vi "circle center from three points.vi"(9 "z plus":cdb, 10 "z zero":cdb, 11 "z minus":cdb) -> (1 "radius":dbl, 2 "z inf":cdb, 3 "z center":cdb)   [LabVIEW 2015]
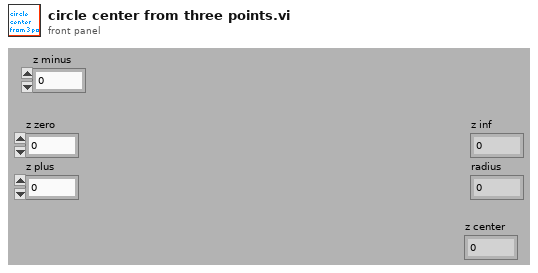
[diagram p1: front panel]
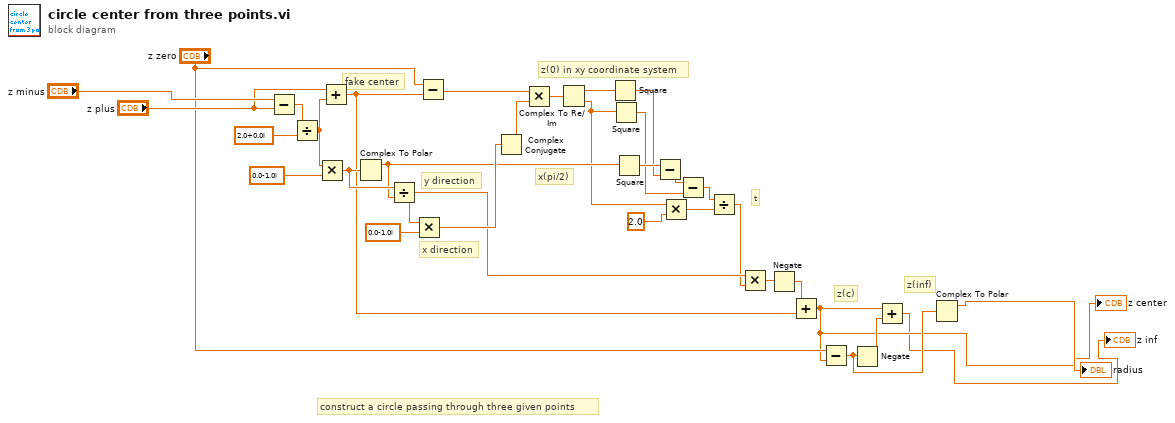
[diagram p0: block diagram]
diagram:
  # "z(inf)"
  # "z(c)"
  # "t"
  # "x(pi/2)"
  # "z(0) in xy coordinate system"
  # "x direction"
  # "y direction"
  # "fake center"
  # "construct a circle passing through three given points"
  n1 = Subtract(x="z minus", y="z plus") -> (x-y=w33:cdb)
  n2 = Divide(x=w33, y=cdb 2.0+0.0i) -> (x/y=w31:cdb)
  n3 = Multiply(x=w31, y=cdb 0.0-1.0i) -> (x*y=w28:cdb)
  n4 = Add(x="z plus", y=w31) -> (x+y=w9:cdb)
  n5 = Complex To Polar(r * e^(i*theta)=w28) -> (r=w23:dbl)  [unwired: 1 out]
  n6 = Divide(x=w28, y=w23) -> (x/y=w13:cdb)
  n7 = Multiply(x=w13, y=cdb 0.0-1.0i) -> (x*y=w27:cdb)
  n8 = Subtract(x="z zero", y=w9) -> (x-y=w25:cdb)
  n9 = Complex Conjugate(1:w27) -> (0:w26:cdb)
  n10 = Multiply(x=w25, y=w26) -> (x*y=w24:cdb)
  n11 = Complex To Re/Im(x + iy=w24) -> (x=w21:dbl, y=w16:dbl)
  n12 = Square(x=w21) -> (x^2=w20:dbl)
  n13 = Square(x=w16) -> (x^2=w18:dbl)
  n14 = Square(x=w23) -> (x^2=w22:dbl)
  n15 = Subtract(x=w22, y=w20) -> (x-y=w19:dbl)
  n16 = Multiply(x=w16, y=2.0) -> (x*y=w14:dbl)
  n17 = Subtract(x=w19, y=w18) -> (x-y=w15:dbl)
  n18 = Divide(x=w15, y=w14) -> (x/y=w12:dbl)
  n19 = Multiply(x=w13, y=w12) -> (x*y=w11:cdb)
  n20 = Negate(x=w11) -> (-x=w10:cdb)
  n21 = Add(x=w10, y=w9) -> (x+y=w2:cdb)
  "z center" <- w2
  n22 = Subtract(x="z zero", y=w2) -> (x-y=w7:cdb)
  n23 = Negate(x=w7) -> (-x=w8:cdb)
  n24 = Add(x=w2, y=w8) -> (x+y=→"z inf":cdb)
  n25 = Complex To Polar(r * e^(i*theta)=w7) -> (r=→"radius":dbl)  [unwired: 1 out]
